vi "TestOFFINISH.vi"(8 "error in (no error)":errorcluster, 11 "OFnext":string) -> (0 "error out":errorcluster)   [LabVIEW 2020]
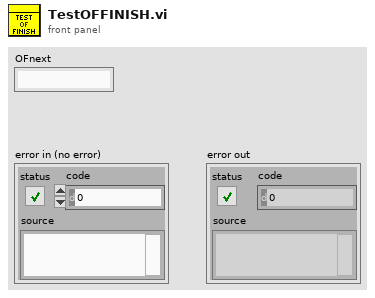
[diagram p1: front panel]
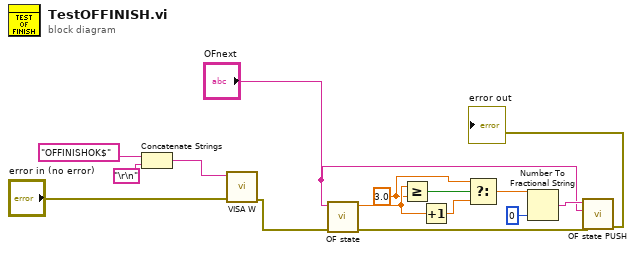
[diagram p0: block diagram]
diagram:
  w9 = 3.0 ("y")
  n1 = Concatenate Strings("OFFINISHOK$" ("buffer d'écriture"), "\r\n") -> (w15:string)
  n2 = call "VISA W.vi"("errin"="error in (no error)", "Chaîne"=w15) -> ("errout"=w14:errorcluster)  [unwired: 9 in]
  n3 = call "OF state.vi"("errin"=w14, "OF"="OFnext") -> ("error out"=w4:errorcluster, "number dbl"=w10:dbl)  [unwired: 7 in, 1 out]
  n4 = Greater Or Equal? ("Supérieur ou égal ?")(x=w10, y=w9) -> (x >= y?=w8:bool)
  n5 = Increment(x=w10) -> (x+1=w11:dbl)
  n6 = Select(t=w9, s=w8, f=w11) -> (s? t:f=w12:dbl)
  n7 = Number To Fractional String ("Nombre en chaîne fractionnaire")(number=w12, precision (6)=i16 0 ("précision (6)")) -> (F-format string=w6:string)  [unwired: 2 in]
  n8 = call "OF state PUSH.vi"("errin"=w4, "OF"="OFnext", "result"=w6) -> ("error out"=→"error out":errorcluster)  [unwired: 8 in]
